vi "Load Calibration from S2P File.vi"(7 "path":string, 8 "error in (no error)":errorcluster, 11 "PathControl in":refnum<class "PathControl.lvclass">) -> (0 "error out":errorcluster, 3 "PathControl out":refnum<class "PathControl.lvclass">)   [LabVIEW 2020, in "PathControl.lvclass"]
uses:
  PathControl.lvclass
  Measurements Specific Paths.ctl
  Paths.ctl
panel:
  in  "Cancel Button":bool
  in  "OK Button":bool
  out "System XY Graph":cluster{dbl[], dbl[]}(graph)
  out "Path":T1
  out "Measurement specific paths":T2=enum."Harmonics"
  in  "S2P File Path":path
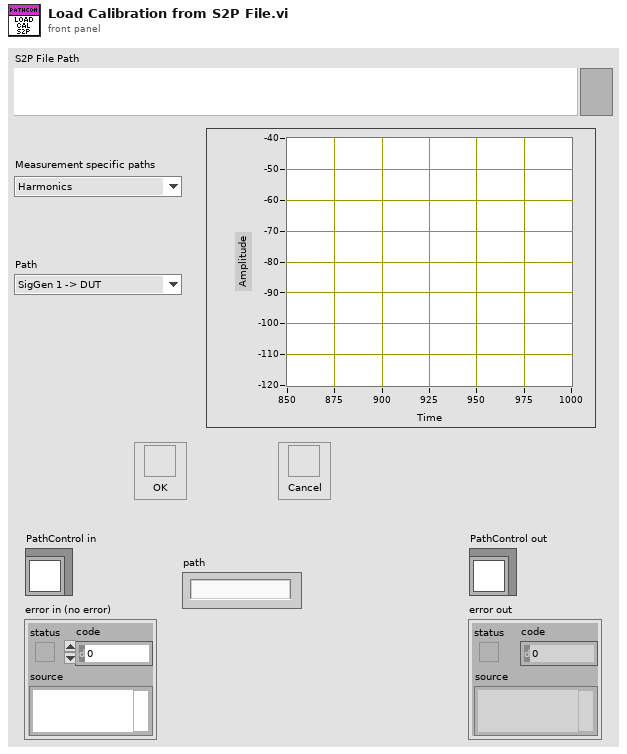
[diagram p1: front panel]
types:
  T1 = typedef "PathControl.lvclass/Paths.ctl" = enum16{"SigGen 1 -> DUT", "SigGen 2 -> DUT", "SigGen 1 -> PM 1", "SigGen 1 -> PM 2", "DUT -> SA", "DUT -> PM 2", "VSG -> DUT", "SigGen 2 -> PM 1", "SigGen 2 -> PM 2"}
  T2 = typedef "PathControl.lvclass/Measurements Specific Paths.ctl" = enum16{"No calibration", "Harmonics", "IMD", "S Parameter", "AM-AM", "MCCW-ACLR", "DC", "LCR", "Power Meter GUI", "RF Power"}
  T3 = typedef "Vector Network Analyzer.lvclass/Sparameter cluster.ctl" = cluster{"Frequency":dbl, "S Parameters":cdb[]}
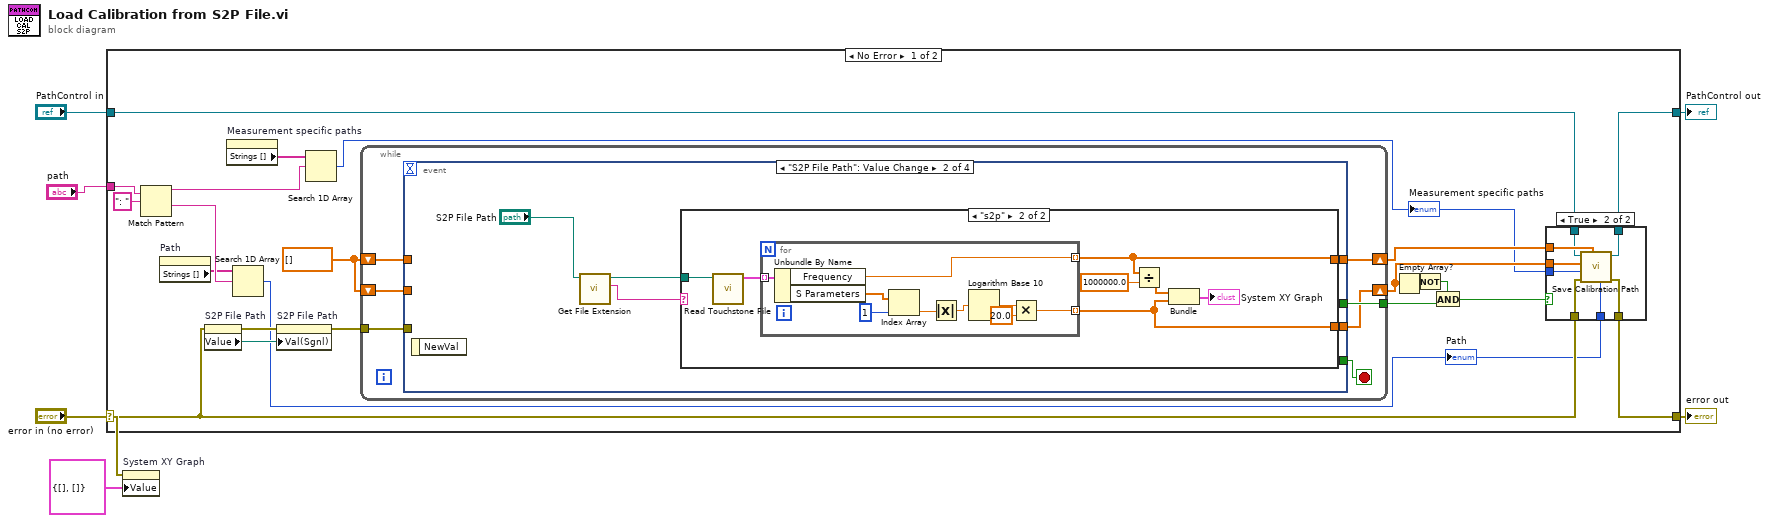
[diagram p0: block diagram]
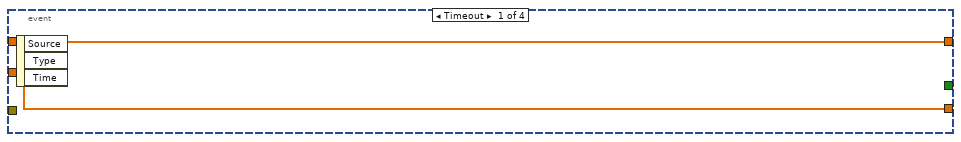
[diagram p3: hidden frame]
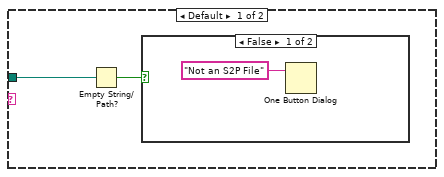
[diagram p4: hidden frame]
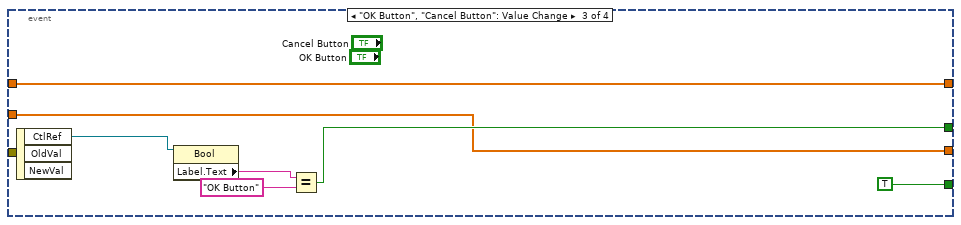
[diagram p6: hidden frame]
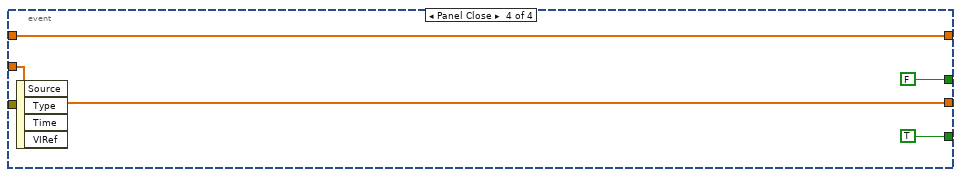
[diagram p7: hidden frame]
diagram:
  n1 = case shown="No Error" "error in (no error)" {
    selector: "error in (no error)" -> [w17 w84]
    tunnel: [w16 w84] -> w6
    tunnel: [w25 w83] -> w4
    tunnel: "PathControl in" -> [w26 w83]
    tunnel: "path" -> [w13 _]
    frame No Error {
      w21 = dbl[] []
      n2 = Match Pattern(string=w13, regular expression=": ") -> (before substring=w11:string, after substring=w10:string)  [unwired: 1 in, 2 out]
      n3 = property on="Path" class="Enum (strict)"() -> ("Strings []"=w9:string[])  [unwired: 2 in, 2 out]
      n4 = property on="S2P File Path" class="Path"(error in=w17) -> (error out=w19:errorcluster, "Value"=w20:path)  [unwired: 1 in, 1 out]
      n5 = property on="Measurement specific paths" class="Enum (strict)"() -> ("Strings []"=w12:string[])  [unwired: 2 in, 2 out]
      n6 = Search 1D Array(1D array=w9, element=w10) -> (index of element=w8:i32)  [unwired: 1 in]
      "Path" <- w8
      n7 = property on="S2P File Path" class="Path"(error in=w19, "Val(Sgnl)"=w20) -> (error out=w18:errorcluster)  [unwired: 1 in, 1 out]
      n8 = Search 1D Array(1D array=w12, element=w11) -> (index of element=w7:i32)  [unwired: 1 in]
      "Measurement specific paths" <- w7
      n9 = while {
        tunnel: w18 -> [w45]
        tunnel: [w43] -> w28
        shift-right: [w42] -> w27
        shift-left: w21 -> [w40]
        shift-right: [w41] -> w24
        shift-left: w21 -> [w39]
        stop <- w44 stop-if-true
        n10 = event shown="[1] \"S2P File Path\": Value Change" {
          selector: _ -> [_ _ _ _]
          dyn-events: _ -> [_ _ _ _]
          timeout: _ -> [_ _ _ _]
          tunnel: w45 -> [_ _ _ _]
          tunnel: [_ _ w75 FALSE] -> w43
          tunnel: [_ _ TRUE TRUE] -> w44
          tunnel: [w47 w50 w73 w82] -> w42
          tunnel: [w46 w49 w72 w81] -> w41
          tunnel: w40 -> [w47 _ w73 w82]
          tunnel: w39 -> [w46 _ w72 w81]
          event Timeout {
            n11 = event-data() -> ()  [unwired: 1 in, 3 out]
          }
          event "S2P File Path": Value Change {
            n12 = event-data() -> ()  [unwired: 1 in, 1 out]
            n13 = call <vilib>:"Get File Extension.vi"("file"="S2P File Path") -> ("lowercase file extension"=w48:string, "dup file"=w51:path)  [unwired: 6 in, 3 out]
            n14 = case shown="\"s2p\"" w48 {
              tunnel: w51 -> [w54 w62]
              tunnel: [_ w56] -> w50
              tunnel: [_ w57] -> w49
              frame Default {
                n15 = Empty String/Path?(string/path=w54) -> (empty?=w53:bool)
                n16 = case shown="False" w53 {
                  frame False {
                    n17 = One Button Dialog(message="Not an S2P File") -> ()  [unwired: 1 in, 1 out]
                  }
                  frame True {
                  }
                }
              }
              frame "s2p" {
                n18 = call "Read Touchstone File.vi"("File Path Control"=w62) -> ("Sparameters"=w61:T3[])  [unwired: 9 in, 1 out]
                n19 = for {
                  tunnel: w61 -> [w71] mode=indexing
                  tunnel: [w64] -> w56 mode=indexing
                  tunnel: [w63] -> w57 mode=indexing
                  n20 = Unbundle By Name(w71) -> ("Frequency"=w64:dbl, "S Parameters"=w70:cdb[])
                  n21 = Index Array(array=w70, index=1) -> (element=w68:cdb)
                  n22 = Absolute Value(x=w68) -> (abs(x)=w67:dbl)
                  n23 = Logarithm Base 10(1:w67) -> (0:w66:dbl)
                  n24 = Multiply(x=w66, y=20.0) -> (x*y=w63:dbl)
                }
                n25 = Divide(x=w56, y=1000000.0) -> (x/y=w58:dbl[])
                n26 = Bundle(w58, w57) -> (→"System XY Graph":cluster{dbl[], dbl[]})  [unwired: 1 in]
              }
            }
          }
          event "OK Button", "Cancel Button": Value Change {
            n27 = event-data() -> ("CtlRef"=w78:refnum<vi>)  [unwired: 1 in, 2 out]
            n28 = property class="Bool"(reference=w78) -> ("Label.Text"=w77:string)  [unwired: 1 in, 2 out]
            n29 = Equal?(x=w77, y="OK Button") -> (x = y?=w75:bool)
          }
          event Panel Close {
            n30 = event-data() -> ()  [unwired: 1 in, 4 out]
          }
        }
      }
      n31 = Empty Array?(array=w24) -> (empty?=w23:bool)
      n32 = Not(x=w23) -> (.not. x?=w22:bool)
      n33 = And(x=w22, y=w28) -> (x .and. y?=w15:bool)
      n34 = case shown="True" w15 {
        tunnel: w27 -> [_ w38]
        tunnel: w26 -> [w29 w37]
        tunnel: [w29 w36] -> w25
        tunnel: w24 -> [_ w35]
        tunnel: w7 -> [_ w34]
        tunnel: w8 -> [_ w33]
        tunnel: w17 -> [w30 w32]
        tunnel: [w30 w31] -> w16
        frame False {
        }
        frame True {
          n35 = call "Save Calibration Path.vi"("Path"=w33, "Frequency"=w38, "Error In"=w32, "Measurement specfic paths"=w34, "Path Loss"=w35, "PathControl in"=w37) -> ("Error Out"=w31:errorcluster, "PathControl out"=w36:refnum<class "PathControl.lvclass">)  [unwired: 4 in]
        }
      }
    }
    frame Error {
    }
  }
  "error out" <- w6
  "PathControl out" <- w4
  n36 = property on="System XY Graph" class="XYGraph (strict)"(error in="error in (no error)", "Value"=cluster{dbl[], sgl[]} {[], []} ("XY Graph")) -> ()  [unwired: 1 in, 2 out]
